vi "Get Referenced Structures Geos.vi"(8 "error in":errorcluster, 10 "SNAME":string, 11 "ParseGDSII in":refnum<class "ParseGDSII.lvclass">) -> (0 "error out":errorcluster, 2 "Geometric":refnum<class "Geometric.lvclass">[](array[class]), 3 "ParseGDSII out":refnum<class "ParseGDSII.lvclass">)   [LabVIEW 2019, in "ParseGDSII.lvclass"]
uses:
  ParseGDSII.lvclass
  Elements/Geometric.lvclass
  731cb9b2-133f-4daa-8872-7e8bee01f7d6.vi/6f0841e4-3cf7-4500-899c-fbea304f5b1f.vi
  40683d7e-b3ac-4d52-9da8-ec4a8002952d.vi/45904b05-565b-4626-aa11-1af00fa7b25d.vi
  <vilib>/Utility/Debug Log/Display.vi
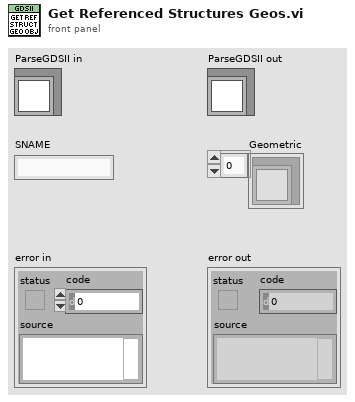
[diagram p1: front panel]
types:
  T1 = cluster{"Record Type":string, "Payload":string, "Parent Index":i32, "First Child Index":i32, "Next Sibling Index":i32}
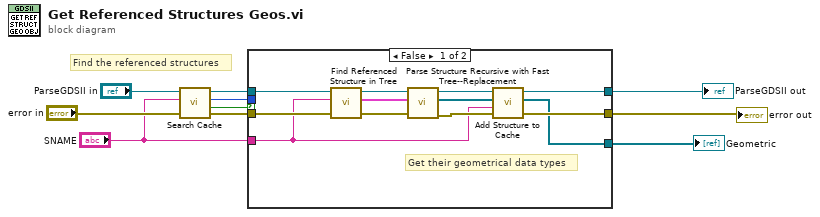
[diagram p0: block diagram]
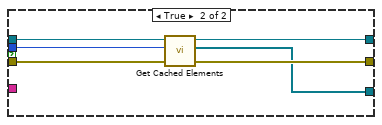
[diagram p2: hidden frame]
diagram:
  # "Find the referenced structures"
  n1 = call "Search Cache.vi"("error in"="error in", "SNAME"="SNAME", "ParseGDSII in"="ParseGDSII in") -> ("error out"=w5:errorcluster, "Found"=w4:bool, "Index"=w3:i32, "ParseGDSII out"=w7:refnum<class "ParseGDSII.lvclass">)  [unwired: 5 in]
  n2 = case shown="False" w4 {
    tunnel: [w22 w28] -> w9
    tunnel: w7 -> [w19 w27]
    tunnel: "SNAME" -> [w11 _]
    tunnel: [w20 w23] -> w10
    tunnel: [w21 w24] -> w2
    tunnel: w5 -> [w18 w25]
    tunnel: w3 -> [_ w26]
    frame False {
      # "Get their geometrical data types"
      n3 = call "Find Referenced Structure in Tree.vi"("error in"=w18, "SNAME"=w11, "ParseGDSII in"=w19) -> ("error out"=w15:errorcluster, "Structure Nodes"=w12:T1, "ParseGDSII out"=w17:refnum<class "ParseGDSII.lvclass">)  [unwired: 6 in]
      n4 = call "Parse Structure Recursive with Fast Tree--Replacement.vi"("error in"=w15, "Node"=w12, "ParseGDSII in"=w17) -> ("error out"=w14:errorcluster, "Geometric Objects"=w13:refnum<class "Geometric.lvclass">[], "ParseGDSII out"=w16:refnum<class "ParseGDSII.lvclass">)  [unwired: 6 in]
      n5 = call "Add Structure to Cache.vi"("error in"=w14, "SREF"=w11, "Geometric In"=w13, "ParseGDSII in"=w16) -> ("error out"=w21:errorcluster, "Geometric Out"=w20:refnum<class "Geometric.lvclass">[], "ParseGDSII out"=w22:refnum<class "ParseGDSII.lvclass">)  [unwired: 5 in]
    }
    frame True {
      n6 = call "Get Cached Elements.vi"("error in"=w25, "Index"=w26, "ParseGDSII in"=w27) -> ("error out"=w24:errorcluster, "Elements"=w23:refnum<class "Geometric.lvclass">[], "ParseGDSII out"=w28:refnum<class "ParseGDSII.lvclass">)  [unwired: 6 in]
    }
  }
  "error out" <- w2
  "ParseGDSII out" <- w9
  "Geometric" <- w10
